vi "Queue Create.vi"(9 "Queue jettl":refnum<class "Queue jettl.lvclass">, 10 "Alias":string, 11 "Base Queue jettl in":refnum<class "Base Queue jettl.lvclass">) -> (3 "Base Queue jettl out":refnum<class "Base Queue jettl.lvclass">)   [LabVIEW 2021, in "jettl.lvlib" / "Base Queue jettl.lvlib" / "Base Queue jettl.lvclass"]
uses:
  Base Queue jettl.lvclass
  Queue jettl/Queue jettl.lvclass
  Msg Strategy/Msg Strategy.lvclass
  Base Queue jettl.lvclass/Base Queue jettl.ctl
  jettl.lvlib
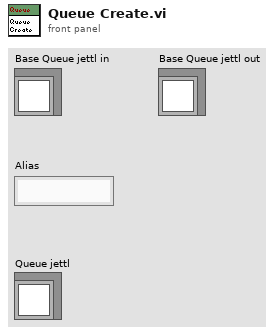
[diagram p1: front panel]
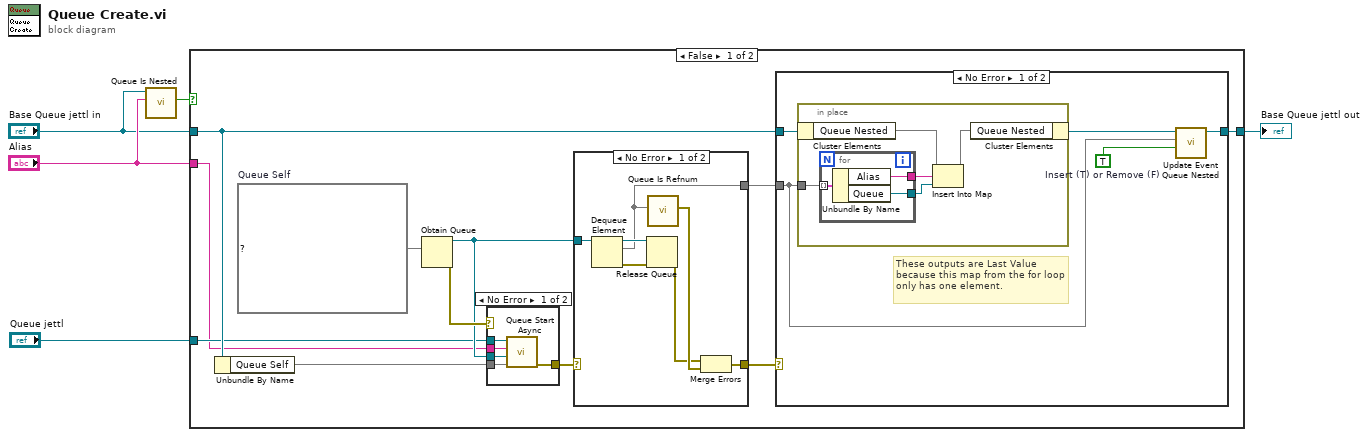
[diagram p0: block diagram]
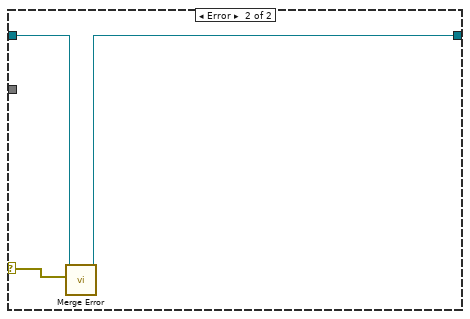
[diagram p4: hidden frame]
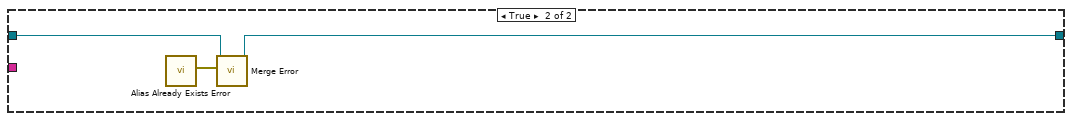
[diagram p5: hidden frame]
diagram:
  n1 = call-dynamic "Queue Is Nested.vi"("Alias"="Alias", "Base Queue jettl in"="Base Queue jettl in") -> ("Queue Is Nested?"=w3:bool)  [unwired: 9 in]
  n2 = case shown="False" w3 {
    tunnel: "Queue jettl" -> [w8 _]
    tunnel: "Base Queue jettl in" -> [w13 w49]
    tunnel: "Alias" -> [w6 _]
    tunnel: [w12 w48] -> w4
    frame False {
      w10 = map{string, refnum<data-value>} {}  # Queue Self
      n3 = Unbundle By Name(w13) -> ("Queue Self"=w14:map{string, refnum<data-value>})
      n4 = Obtain Queue(element data type=w10) -> (queue out=w9:refnum<queue>, error out=w16:errorcluster)  [unwired: 4 in, 1 out]
      n5 = case shown="No Error" w16 {
        selector: w16 -> [_ w30]
        tunnel: [w28 w30] -> w11
        tunnel: w8 -> [w29 _]
        tunnel: w14 -> [w26 _]
        tunnel: w9 -> [w27 _]
        tunnel: w6 -> [w25 _]
        frame No Error {
          n6 = call "Queue Start Async.vi"("Queue Caller"=w26, "Queue of Queue Self"=w27, "Queue Self Alias"=w25, "Queue jettl"=w29) -> ("error out"=w28:errorcluster)  [unwired: 7 in]
        }
        frame Error {
        }
      }
      n7 = case shown="No Error" w11 {
        selector: w11 -> [_ w24]
        tunnel: [w21 w24] -> w15
        tunnel: w9 -> [w18 _]
        tunnel: [w17 _] -> w7
        frame No Error {
          n8 = Dequeue Element(queue=w18) -> (queue out=w22:refnum<queue>, element=w17:map{string, refnum<data-value>}, error out=w23:errorcluster)  [unwired: 2 in, 1 out]
          n9 = Release Queue(queue=w22, error in (no error)=w23) -> (error out=w19:errorcluster)  [unwired: 1 in, 2 out]
          n10 = call "Queue Is Refnum.vi"("Queue Self"=w17) -> ("Error"=w20:errorcluster)  [unwired: 10 in]
          n11 = Merge Errors(w19, w20) -> (w21:errorcluster)
        }
        frame Error {
        }
      }
      n12 = case shown="No Error" w15 {
        selector: w15 -> [_ w44]
        tunnel: w13 -> [w35 w46]
        tunnel: [w33 w45] -> w12
        tunnel: w7 -> [w32 _]
        frame No Error {
          w31 = TRUE  # Insert (T) or Remove (F)
          # "These outputs are Last Value because this map from the for loop only has one element."
          n13 = in-place {
            in-place-border: w32 -> [w38]
            n14 = in-place-cluster #1(w35) -> ("Queue Nested"=w40:map{string, refnum<data-value>})
            n15 = for {
              tunnel: w38 -> [w43] mode=indexing
              tunnel: [w42] -> w37
              tunnel: [w41] -> w36
              n16 = Unbundle By Name(w43) -> ("Alias"=w42:string, "Queue"=w41:refnum<data-value>)
            }
            n17 = Insert Into Map(map in=w40, key=w37, value=w36) -> (map out=w39:map{string, refnum<data-value>})  [unwired: 2 out]
            n18 = in-place-cluster #1("Queue Nested"=w39) -> (w34:refnum<class "Base Queue jettl.lvclass">)
          }
          n19 = call "Update Event Queue Nested.vi"("Insert (T) or Remove (F)"=w31, "Queue Nested"=w32, "Base Queue jettl in"=w34) -> ("Base Queue jettl out"=w33:refnum<class "Base Queue jettl.lvclass">)  [unwired: 8 in]
        }
        frame Error {
          n20 = call-dynamic "Merge Error.vi"("Error"=w44, "Base Queue jettl in"=w46) -> ("Base Queue jettl out"=w45:refnum<class "Base Queue jettl.lvclass">)  [unwired: 9 in]
        }
      }
    }
    frame True {
      n21 = call "Alias Already Exists Error.vi"() -> ("Error"=w47:errorcluster)  [unwired: 11 in]
      n22 = call-dynamic "Merge Error.vi"("Error"=w47, "Base Queue jettl in"=w49) -> ("Base Queue jettl out"=w48:refnum<class "Base Queue jettl.lvclass">)  [unwired: 9 in]
    }
  }
  "Base Queue jettl out" <- w4
